vi "GOOP_CreateClassFromTemplate.vi"(0 "Application in":refnum<vi>, 2 "ClassFolder":path, 3 "TeplateClassFolder":path, 5 "error in (no error)":errorcluster, 6 "ClassName":string) -> (10 "TemplateParentName":string, 12 "NewClassRef":refnum<vi>, 13 "TemplateClassVersionString":string, 14 "TemplateClassRef":refnum<vi>, 16 "TemplateClassConstructorPath(*Create, *Init)":path, 17 "NewClassPath":path, 18 "TemplateClassPath":path, 19 "error out":errorcluster)   [LabVIEW 2016]
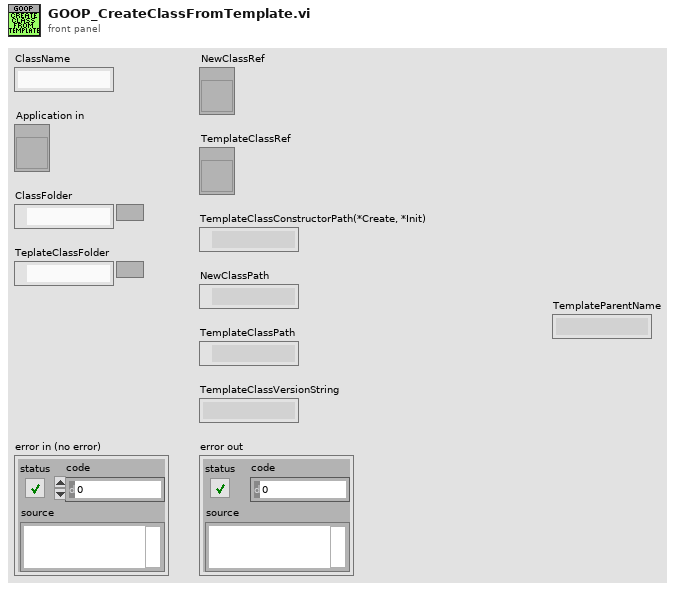
[diagram p1: front panel]
types:
  T1 = enum16{"Remove Parent's Inheritance before cloning", "Don't Remove Parent's Inheritance before cloning", "Create a Template Copy where we remove the Parents inheritance on"}
  T2 = cluster{"Major":u16, "Minor":u16, "Fix":u16, "Build":u16}
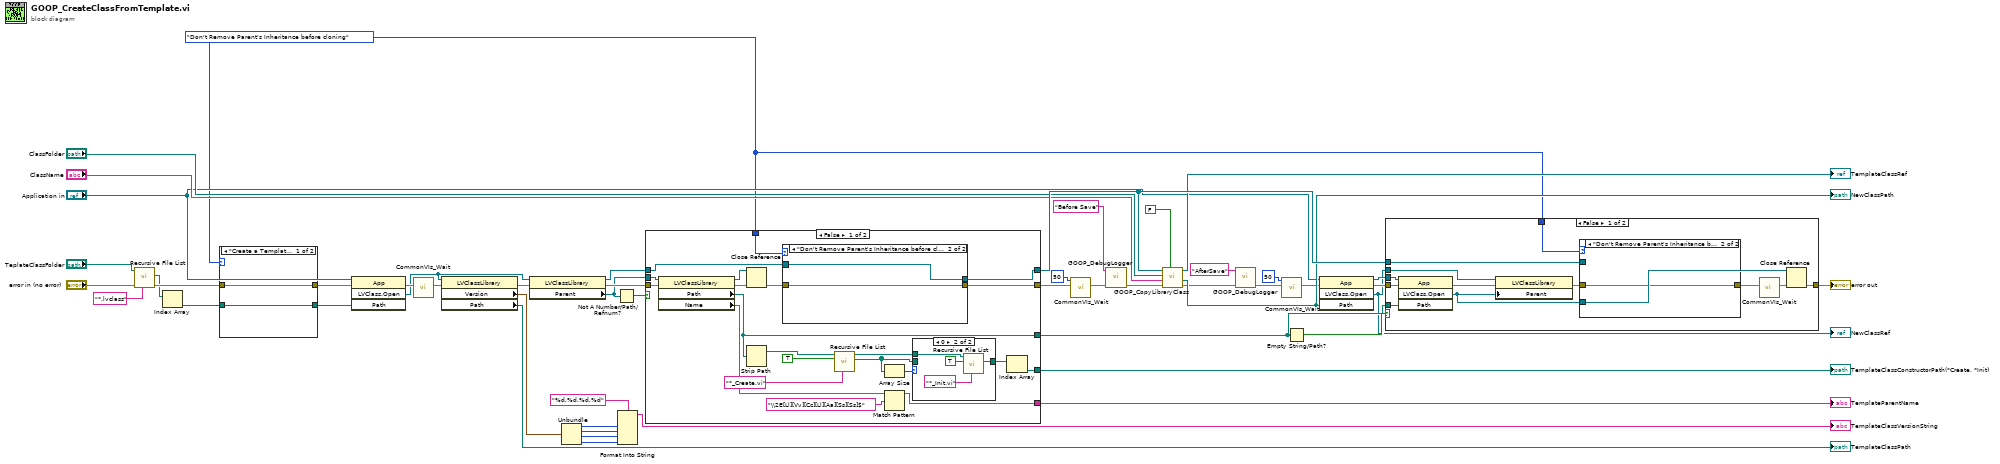
[diagram p0: block diagram]
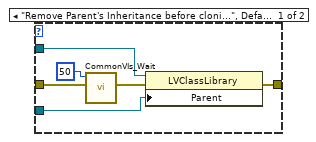
[diagram p3: hidden frame]
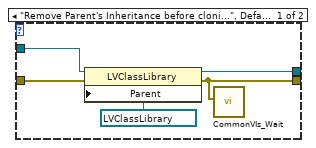
[diagram p5: hidden frame]
diagram:
  w1 = T1."Don't Remove Parent's Inheritance before cloning" ("CreationOption")
  n1 = call <vilib>:"Recursive File List.vi"("pattern"="*.lvclass", "error in (no error)"="error in (no error)", "Folder Path"="TeplateClassFolder") -> ("error out"=w31:errorcluster, "All Files in Dir"=w6:path[])  [unwired: 4 in, 3 out]
  n2 = Index Array(array=w6) -> (element=w7:path)  [unwired: 1 in]
  n3 = case shown="\"Create a Template Copy where we remove the Parents inheritance on\"" w1 {
    tunnel: w31 -> [w52 w54]
    tunnel: w7 -> [w51 w53]
    tunnel: [w52 w54] -> w3
    tunnel: [w51 w53] -> w2
    frame "Create a Template Copy where we remove the Parents inheritance on" {
    }
    frame Default {
    }
  }
  n4 = invoke class="App" method="LVClass.Open"(reference="Application in", error in=w3, "Path"=w2) -> (error out=w35:errorcluster, "LVClass.Open"=w23:refnum<vi>)  [unwired: 1 in, 2 out]
  n5 = call <resource>:"CommonVIs_Wait.vi"("error in"=w35) -> ("error out"=w34:errorcluster)  [unwired: 9 in]
  n6 = property class="LVClassLibrary"(reference=w23, error in=w34) -> (error out=w22:errorcluster, "Version"=w10:T2, "Path"=→"TemplateClassPath":path)  [unwired: 1 out]
  n7 = property class="LVClassLibrary"(reference=w23, error in=w22) -> (reference out=w18:refnum<vi>, error out=w26:errorcluster, "Parent"=w25:refnum<vi>)
  n8 = Unbundle(w10) -> ("Major"=w12:u16, "Minor"=w13:u16, "Fix"=w14:u16, "Build"=w15:u16)
  n9 = Not A Number/Path/Refnum?(number/path/refnum=w25) -> (NaN/Path/Refnum?=w27:bool)
  n10 = Format Into String(format string="%d.%d.%d.%d", w12, w13, w14, w15) -> (resulting string=→"TemplateClassVersionString":string)  [unwired: 2 in, 1 out]
  n11 = case shown="False" w27 {
    tunnel: w18 -> [w72 w88]
    tunnel: [w71 w88] -> w50
    tunnel: [w59 w89] -> w36
    tunnel: [w68 _] -> w24
    tunnel: w25 -> [w66 _]
    tunnel: w26 -> [w65 w89]
    tunnel: [w64 _] -> w28
    tunnel: [w56 _] -> w4
    tunnel: w1 -> [w55 _]
    frame False {
      n12 = property class="LVClassLibrary"(reference=w66, error in=w65) -> (reference out=w74:refnum<vi>, error out=w75:errorcluster, "Path"=w64:path, "Name"=w57:string)
      n13 = Close Reference(reference=w74, error in (no error)=w75) -> (error out=w73:errorcluster)
      n14 = Strip Path(path=w64) -> (stripped path=w67:path)  [unwired: 1 out]
      n15 = case shown="\"Don't Remove Parent's Inheritance before cloning\"" w55 {
        tunnel: w73 -> [w80 w82]
        tunnel: w72 -> [w79 w81]
        tunnel: [w78 w81] -> w71
        tunnel: [w77 w82] -> w59
        frame "Remove Parent's Inheritance before cloning", Default {
          n16 = property class="LVClassLibrary"(reference=w79, error in=w80, "Parent"=refnum<vi> refnum ("Parent Class")) -> (reference out=w78:refnum<vi>, error out=w77:errorcluster)
          n17 = call <resource>:"CommonVIs_Wait.vi"("error in"=w77) -> ()  [unwired: 9 in, 1 out]
        }
        frame "Don't Remove Parent's Inheritance before cloning" {
        }
      }
      n18 = call <vilib>:"Recursive File List.vi"("pattern"="*_Create.vi", "Treat LLBs as Folders?"=TRUE, "Folder Path"=w67) -> ("All Files in Dir"=w60:path[], "dup Folder Path"=w61:path)  [unwired: 4 in, 3 out]
      n19 = Array Size(array=w60) -> (size(s)=w63:i32)
      n20 = Match Pattern(string=w57, regular expression="\\2E[Ll][Vv][Cc][Ll][Aa][Ss][Ss]$") -> (before substring=w56:string)  [unwired: 1 in, 3 out]
      n21 = case shown="0" w63 {
        tunnel: w60 -> [w83 _]
        tunnel: [w83 w84] -> w62
        tunnel: w61 -> [_ w85]
        frame Default {
        }
        frame 0 {
          n22 = call <vilib>:"Recursive File List.vi"("pattern"="*_Init.vi", "Treat LLBs as Folders?"=TRUE, "Folder Path"=w85) -> ("All Files in Dir"=w84:path[])  [unwired: 4 in, 4 out]
        }
      }
      n23 = Index Array(array=w62) -> (element=w68:path)  [unwired: 1 in]
    }
    frame True {
    }
  }
  "TemplateClassConstructorPath(*Create, *Init)" <- w24
  "TemplateParentName" <- w4
  n24 = call <resource>:"CommonVIs_Wait.vi"("error in"=w36, "Wait(150ms)"=u32 50) -> ("error out"=w39:errorcluster)  [unwired: 8 in]
  n25 = call <resource>:"GOOP_DebugLogger.vi"("error in (no error)"=w39, "State"="Before Save") -> ("error out"=w44:errorcluster)  [unwired: 7 in, 2 out]
  n26 = call <resource>:"GOOP_CopyLibraryClass.vi"("ManualCopy"=FALSE, "error in"=w44, "New Name"="ClassName", "Path"="ClassFolder", "LVClassIn"=w50) -> ("error out"=w45:errorcluster, "New Lib Path"=w46:path, "LVClassOut"=→"TemplateClassRef":refnum<vi>)  [unwired: 4 in]
  "NewClassPath" <- w46
  n27 = call <resource>:"GOOP_DebugLogger.vi"("error in (no error)"=w45, "State"="AfterSave") -> ("error out"=w41:errorcluster)  [unwired: 7 in, 2 out]
  n28 = call <resource>:"CommonVIs_Wait.vi"("error in"=w41, "Wait(150ms)"=u32 50) -> ("error out"=w33:errorcluster)  [unwired: 8 in]
  n29 = Empty String/Path?(string/path=w28) -> (empty?=w29:bool)
  n30 = invoke class="App" method="LVClass.Open"(reference="Application in", error in=w33, "Path"=w46) -> (reference out=w20:refnum<vi>, error out=w21:errorcluster, "LVClass.Open"=w19:refnum<vi>)  [unwired: 1 in, 1 out]
  "NewClassRef" <- w19
  n31 = case shown="False" w29 {
    tunnel: w19 -> [w101 _]
    tunnel: w20 -> [w100 _]
    tunnel: w21 -> [w99 w109]
    tunnel: [w98 w109] -> w32
    tunnel: w28 -> [w97 _]
    tunnel: w50 -> [w94 _]
    tunnel: w1 -> [w90 _]
    frame False {
      n32 = invoke class="App" method="LVClass.Open"(reference=w100, error in=w99, "Path"=w97) -> (error out=w96:errorcluster, "LVClass.Open"=w93:refnum<vi>)  [unwired: 1 in, 2 out]
      n33 = property class="LVClassLibrary"(reference=w101, error in=w96, "Parent"=w93) -> (error out=w91:errorcluster)  [unwired: 1 out]
      n34 = case shown="\"Don't Remove Parent's Inheritance before cloning\", \"Create a Template Copy where we remove the Parents inheritance on\"" w90 {
        tunnel: w94 -> [w107 _]
        tunnel: w93 -> [w106 _]
        tunnel: [w105 w108] -> w92
        tunnel: w91 -> [w104 w108]
        frame "Remove Parent's Inheritance before cloning", Default {
          n35 = call <resource>:"CommonVIs_Wait.vi"("error in"=w104, "Wait(150ms)"=u32 50) -> ("error out"=w103:errorcluster)  [unwired: 8 in]
          n36 = property class="LVClassLibrary"(reference=w107, error in=w103, "Parent"=w106) -> (error out=w105:errorcluster)  [unwired: 1 out]
        }
        frame "Don't Remove Parent's Inheritance before cloning", "Create a Template Copy where we remove the Parents inheritance on" {
        }
      }
      n37 = call <resource>:"CommonVIs_Wait.vi"("error in"=w92) -> ("error out"=w95:errorcluster)  [unwired: 9 in]
      n38 = Close Reference(reference=w93, error in (no error)=w95) -> (error out=w98:errorcluster)
    }
    frame True {
    }
  }
  "error out" <- w32
